vi "Ball stop.vi"() -> ()   [LabVIEW 2019]
panel:
  out "encoder greater than Minimum angle":bool
  out "encoder les than forewards angle":bool
  out "encoder les than target":bool
  in  "Speed":dbl=0.5
  in  "Minimum angle":dbl
  in  "Backwards":bool
  in  "Encoder simulation":dbl(knob) scale=0.0..10.0
  out "Angle Target":u32
  out "Encoder angle":u32
  in  "Forwards angle":dbl
  in  "Finish":bool
  in  "Forwards":bool
  out "Output":dbl
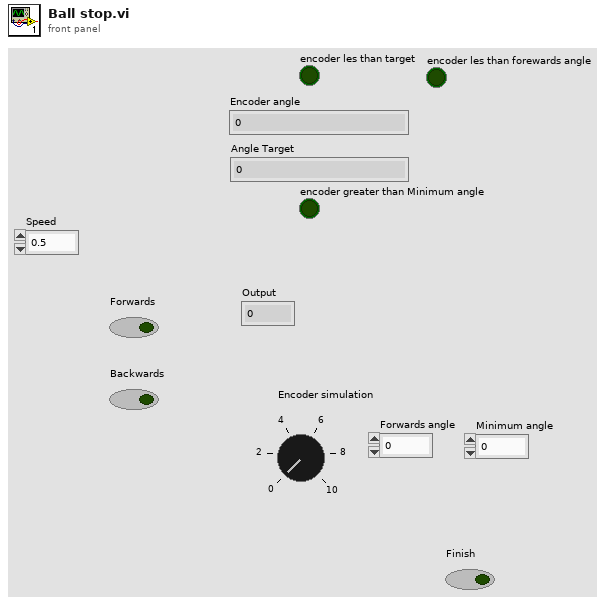
[diagram p1: front panel]
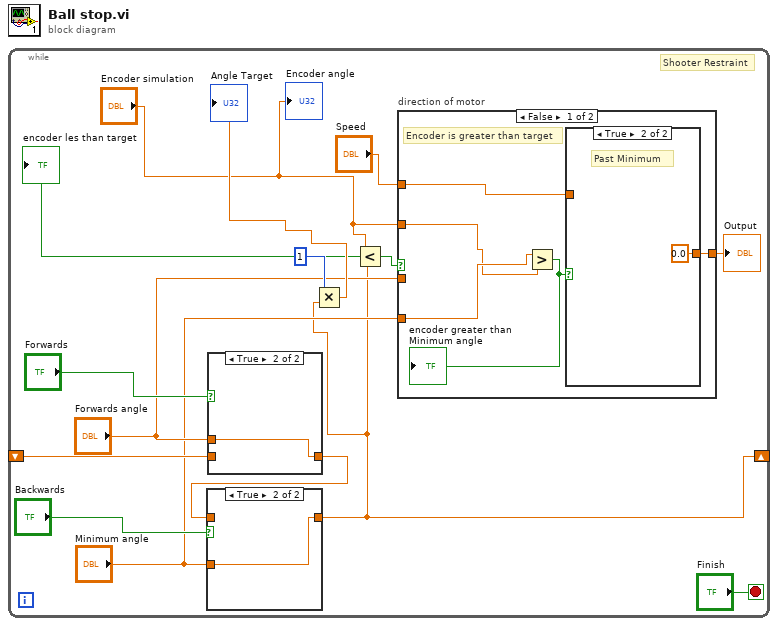
[diagram p0: block diagram]
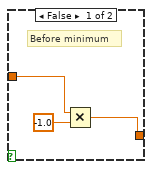
[diagram p2: hidden frame]
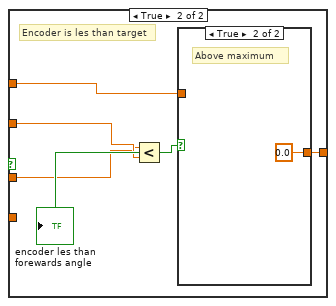
[diagram p3: hidden frame]
diagram:
  n1 = while {
    shift-right: [w2] -> _
    shift-left: _ -> [w9]
    stop <- "Finish" stop-if-true
    # "Shooter Restraint"
    n2 = case shown="True" "Forwards" {
      tunnel: [w33 w34] -> w10
      tunnel: w9 -> [w33 _]
      tunnel: "Forwards angle" -> [_ w34]
      frame False {
      }
      frame True {
      }
    }
    n3 = case shown="True" "Backwards" {
      tunnel: [w31 w32] -> w2
      tunnel: w10 -> [w31 _]
      tunnel: "Minimum angle" -> [_ w32]
      frame False {
      }
      frame True {
      }
    }
    n4 = Multiply(x=u32 1, y=w2) -> (x*y=→"Angle Target":dbl)
    n5 = Less?(x="Encoder simulation", y=w2) -> (x < y?=w1:bool)
    "encoder les than target" <- w1
    n6 = case "direction of motor" shown="False" w1 {
      tunnel: "Encoder simulation" -> [w15 w25]
      tunnel: "Forwards angle" -> [_ w24]
      tunnel: "Minimum angle" -> [w16 _]
      tunnel: [w18 w27] -> w4
      tunnel: "Speed" -> [w17 w26]
      frame False {
        # "Encoder is greater than target"
        n7 = Greater?(x=w16, y=w15) -> (0:w19:bool)
        "encoder greater than Minimum angle" <- w19
        n8 = case shown="True" w19 {
          tunnel: [w20 0.0] -> w18
          tunnel: w17 -> [w21 _]
          frame False {
            # "Before minimum"
            n9 = Multiply(x=w21, y=-1.0) -> (x*y=w20:dbl)
          }
          frame True {
            # "Past Minimum"
          }
        }
      }
      frame True {
        # "Encoder is les than target"
        n10 = Less?(x=w24, y=w25) -> (x < y?=w28:bool)
        "encoder les than forewards angle" <- w28
        n11 = case shown="True" w28 {
          tunnel: [w29 0.0 ("Output")] -> w27
          tunnel: w26 -> [w29 _]
          frame False {
            # "Before Maximum"
          }
          frame True {
            # "Above maximum"
          }
        }
      }
    }
    "Output" <- w4
    "Encoder angle" <- "Encoder simulation"
  }
